vi "run VI with parameters.vi"(7 "reentrant? (T)":bool=TRUE, 8 "error in":errorcluster, 9 "data":variant[](array[variant]), 10 "terminals":string[](array[string]), 11 "VI path":path) -> (0 "error out":errorcluster)   [LabVIEW 2013]
doc: "Runs a VI using the run VI method, providing it with any input parameters. This instance accepts a VI path."
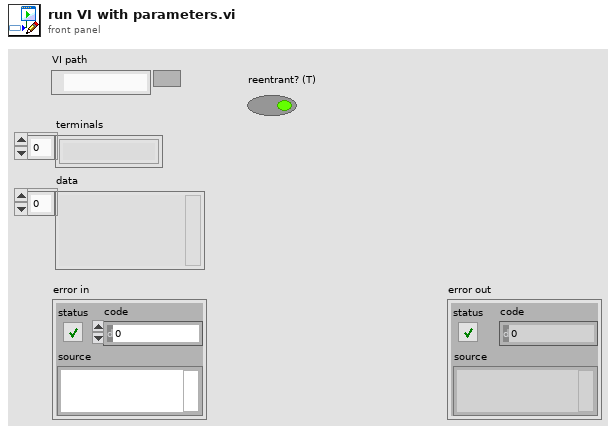
[diagram p1: front panel]
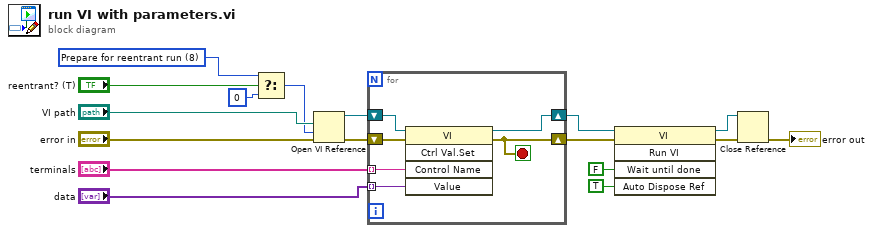
[diagram p0: block diagram]
diagram:
  w3 = 8 items=["Prepare for reentrant run"=8, "Enable simultaneous calls on reentrant VIs"=64, "Prepare to call and forget"=128, "Prepare to call and collect"=256, "Reentrant call and forget"=192, "Reentrant call and collect"=320] ("VI Server Options")
  n1 = Select(t=w3, s="reentrant? (T)", f=0 ("options")) -> (s? t:f=w1:i32)
  n2 = Open VI Reference(vi path="VI path", options=w1, error in (no error)="error in") -> (vi reference=w14:refnum<vi>, error out=w15:errorcluster)  [unwired: 3 in]
  n3 = for {
    shift-right: [w22] -> w10
    shift-left: w15 -> [w23]
    shift-right: [w21] -> w11
    shift-left: w14 -> [w20]
    tunnel: "terminals" -> [w19] mode=indexing
    tunnel: "data" -> [w18] mode=indexing
    stop <- w22 stop-if-true
    n4 = invoke class="VI" method="Ctrl Val.Set"(reference=w20, error in=w23, "Control Name"=w19, "Value"=w18) -> (reference out=w21:refnum<vi>, error out=w22:errorcluster)  [unwired: 1 in, 3 out]
  }
  n5 = invoke class="VI" method="Run VI"(reference=w11, error in=w10, "Wait until done"=FALSE ("Wait Until Done"), "Auto Dispose Ref"=TRUE ("Auto Dispose Reference")) -> (reference out=w6:refnum<vi>, error out=w7:errorcluster)  [unwired: 1 in, 3 out]
  n6 = Close Reference(reference=w6, error in (no error)=w7) -> (error out=→"error out":errorcluster)
